vi "Parse Axis Number.vi"(5 "Y Axis Channel":i32, 7 "X Axis Channel":i32, 9 "Channel":i32) -> (1 "Axis":T1)   [LabVIEW 2017, in "XYStage.KIM101.lvclass"]
uses:
  XYStage.KIM101.lvclass
  XYStage/Typedefs/XYStage.Axis--Enum.ctl
  XYStage/XYStage.lvclass
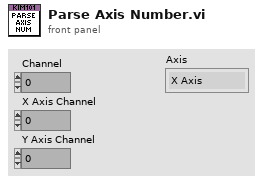
[diagram p1: front panel]
types:
  T1 = typedef "XYStage.lvclass/XYStage.Axis--Enum.ctl" = enum16{"X Axis", "Y Axis", "Undefined"}
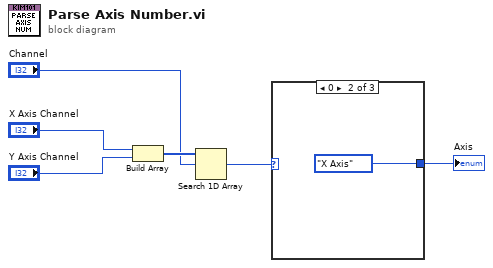
[diagram p0: block diagram]
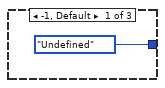
[diagram p2: hidden frame]
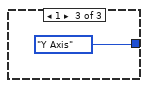
[diagram p3: hidden frame]
diagram:
  n1 = Build Array("X Axis Channel", "Y Axis Channel") -> (w4:i32[])
  n2 = Search 1D Array(1D array=w4, element="Channel") -> (index of element=w2:i32)  [unwired: 1 in]
  n3 = case shown="0" w2 {
    tunnel: [XYStage.Axis--Enum."Undefined" ("Axis") XYStage.Axis--Enum."X Axis" ("Axis") XYStage.Axis--Enum."Y Axis" ("Axis")] -> w1
    frame -1, Default {
    }
    frame 0 {
    }
    frame 1 {
    }
  }
  "Axis" <- w1
